vi "command_file__duration.vi"() -> ()   [LabVIEW 2019]
uses:
  Global Variables/global.vi
  Global Variables/Data_Display_global.vi
  Instrument_Setup.vi
panel:
  out "Remaining measurement time of row":string
  out "Measurement ends:":string
  out "Remaining measurement time":string
  out "Measurement Time":string
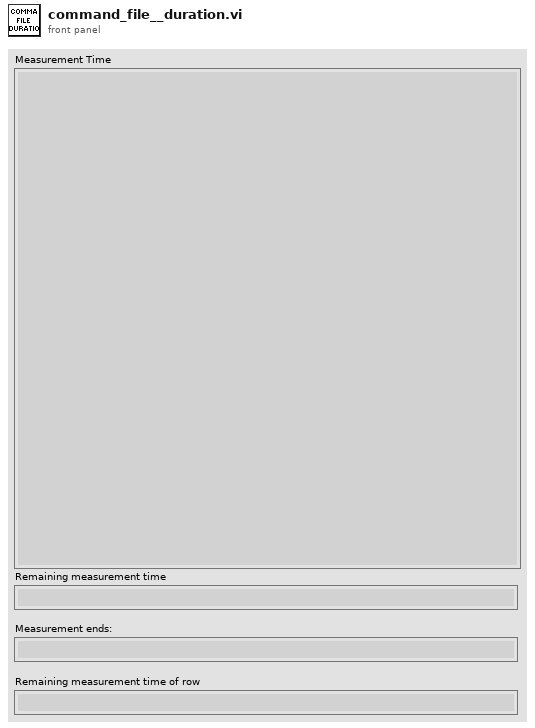
[diagram p1: front panel]
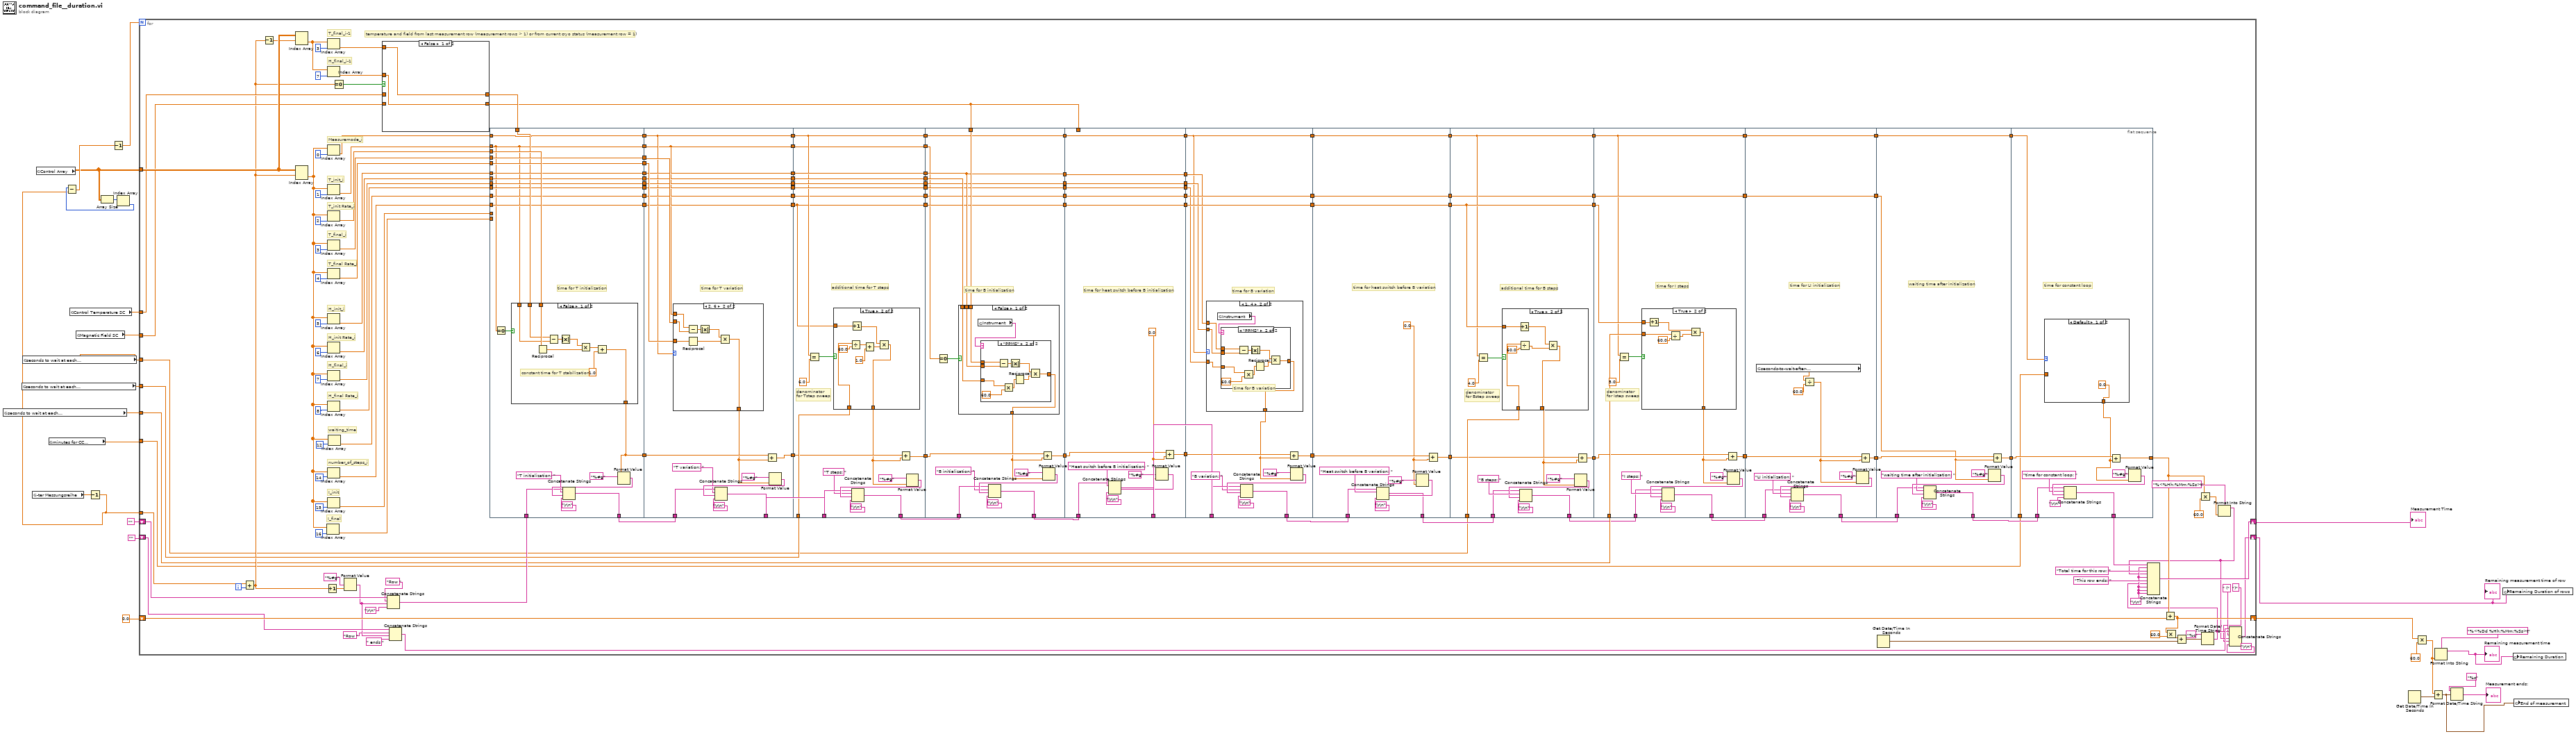
[diagram p0: block diagram]
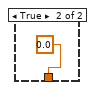
[diagram p3: hidden frame]
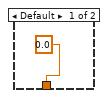
[diagram p4: hidden frame]
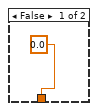
[diagram p5: hidden frame]
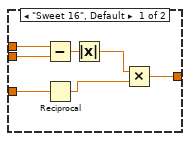
[diagram p6: hidden frame]
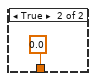
[diagram p7: hidden frame]
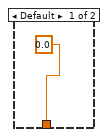
[diagram p8: hidden frame]
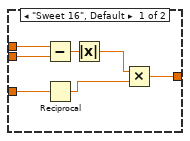
[diagram p9: hidden frame]
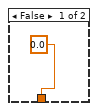
[diagram p10: hidden frame]
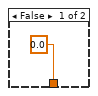
[diagram p11: hidden frame]
diagram:
  n1 = global read "Instrument_Setup.vi" "seconds to wait at each\ncurrent step in a I-step sweep"() -> (w7:dbl)
  n2 = global read "Instrument_Setup.vi" "seconds to wait at each\nfield step in a step sweep"() -> (w8:dbl)
  n3 = global read "Instrument_Setup.vi" "seconds to wait at each\nfield step in a step sweep"() -> (w9:dbl)
  n4 = global read "global.vi" "-ter Messungsreihe"() -> (w4:dbl)
  n5 = global read "global.vi" "Control Array"() -> (w14:dbl[][])
  n6 = global read "Instrument_Setup.vi" "minutes for CC\nto run"() -> (w6:dbl)
  n7 = global read "Data_Display_global.vi" "Control Temperature SC"() -> (w11:dbl)
  n8 = global read "Data_Display_global.vi" "Magnetic Field SC"() -> (w10:dbl)
  n9 = Decrement(x=w4) -> (x-1=w5:dbl)
  n10 = Array Size(array=w14) -> (size(s)=w27:i32[])
  n11 = Index Array(array=w27) -> (element=w22:i32)  [unwired: 1 in]
  n12 = Subtract(x=w22, y=w5) -> (x-y=w23:dbl)
  n13 = Decrement(x=w23) -> (x-1=w26:dbl)
  n14 = for {
    N: w26 -> [_]
    tunnel: w14 -> [w154]
    shift-right: [w130] -> w24
    shift-left: "" -> [w123]
    tunnel: w11 -> [w147]
    tunnel: w10 -> [w146]
    tunnel: w9 -> [w96]
    tunnel: w5 -> [w156]
    tunnel: w8 -> [w135]
    tunnel: w7 -> [w91]
    shift-right: [w71] -> w19
    shift-left: 0.0 -> [w76]
    tunnel: w6 -> [w42]
    shift-right: [w35] -> w2
    shift-left: "" -> [w39]
    i -> [w155]
    w68 = "\r\n"
    # "waiting_time"
    # "I_final"
    # "I_init"
    # "temperature and field from last measurement row (measurement rows > 1) or from current cryo status (measurement row = 1)"
    # "H_final_i-1"
    # "T_final_i-1"
    # "Measuremode_i"
    # "number_of_steps_i"
    # "H_final Rate_i"
    # "H_final_i"
    # "H_init Rate_i"
    # "H_init_i"
    # "T_final Rate_i"
    # "T_final_i"
    # "T_init Rate_i"
    # "T_init_i"
    n15 = Add(x=w156, y=w155) -> (x+y=w121:dbl)
    n16 = Decrement(x=w121) -> (x-1=w153:dbl)
    n17 = Index Array(array=w154, index (row)=w153) -> (element=w150:dbl[])  [unwired: 1 in]
    n18 = Index Array(array=w154, index (row)=w121) -> (element=w60:dbl[])  [unwired: 1 in]
    n19 = Increment(x=w121) -> (x+1=w120:dbl)
    n20 = Index Array(array=w60, index=16) -> (element=w92:dbl)
    n21 = Index Array(array=w150, index=3) -> (element=w149:dbl)
    n22 = Index Array(array=w150, index=7) -> (element=w148:dbl)
    n23 = Index Array(array=w60, index=0) -> (element=w157:dbl)
    n24 = Index Array(array=w60, index=1) -> (element=w172:dbl)
    n25 = Index Array(array=w60, index=2) -> (element=w171:dbl)
    n26 = Index Array(array=w60, index=3) -> (element=w170:dbl)
    n27 = Index Array(array=w60, index=4) -> (element=w169:dbl)
    n28 = Index Array(array=w60, index=5) -> (element=w168:dbl)
    n29 = Index Array(array=w60, index=6) -> (element=w167:dbl)
    n30 = Index Array(array=w60, index=7) -> (element=w166:dbl)
    n31 = Index Array(array=w60, index=8) -> (element=w165:dbl)
    n32 = Index Array(array=w60, index=14) -> (element=w160:dbl)
    n33 = Index Array(array=w60, index=15) -> (element=w93:dbl)
    n34 = Index Array(array=w60, index=12) -> (element=w59:dbl)
    n35 = Equal To 0?(x=w121) -> (x = 0?=w145:bool)
    n36 = Format Value(format string="%#g", value (0)=w120) -> (output string=w37:string)  [unwired: 1 in]
    n37 = case shown="False" w145 {
      tunnel: w149 -> [w181 _]
      tunnel: w148 -> [w182 _]
      tunnel: w147 -> [_ w184]
      tunnel: w146 -> [_ w183]
      tunnel: [w181 w184] -> w144
      tunnel: [w182 w183] -> w109
      frame False {
      }
      frame True {
      }
    }
    n38 = Concatenate Strings(w123, "Row ", w37, "\r\n") -> (w122:string)
    n39 = Concatenate Strings(w39, "Row ", w37, " ends ") -> (w32:string)
    n40 = flat-sequence {
      tunnel: w172 -> [w185]
      tunnel: w171 -> [w204]
      tunnel: w122 -> [w191]
      tunnel: [w202] -> w161
      tunnel: w170 -> [w199]
      tunnel: w169 -> [w198]
      tunnel: w168 -> [w197]
      tunnel: w167 -> [w196]
      tunnel: w166 -> [w193]
      tunnel: w165 -> [w192]
      tunnel: [w185] -> w164
      tunnel: [w199] -> w163
      tunnel: [w198] -> w162
      tunnel: w160 -> [w194]
      tunnel: [w197] -> w159
      tunnel: [w196] -> w158
      tunnel: w157 -> [w186]
      tunnel: w144 -> [w195]
      tunnel: [w186] -> w136
      tunnel: [w194] -> w133
      tunnel: [w193] -> w129
      tunnel: [w192] -> w124
      tunnel: w93 -> [_]
      tunnel: w92 -> [_]
      tunnel: [w189] -> w86
      tunnel: w59 -> [w188]
      tunnel: [w188] -> w49
      tunnel: w164 -> [w215]
      tunnel: w163 -> [w230]
      tunnel: w162 -> [w229]
      tunnel: [w228] -> w132
      tunnel: w161 -> [w222]
      tunnel: w159 -> [w227]
      tunnel: [w227] -> w141
      tunnel: [w226] -> w139
      tunnel: w158 -> [w226]
      tunnel: [w216] -> w137
      tunnel: w136 -> [w216]
      tunnel: [w225] -> w134
      tunnel: w133 -> [w225]
      tunnel: w129 -> [w224]
      tunnel: [w224] -> w127
      tunnel: [w223] -> w125
      tunnel: w124 -> [w223]
      tunnel: w86 -> [w220]
      tunnel: [w218] -> w85
      tunnel: [w217] -> w50
      tunnel: w49 -> [w217]
      tunnel: [w215] -> w40
      tunnel: w141 -> [w261]
      tunnel: [w261] -> w140
      tunnel: w139 -> [w260]
      tunnel: [w260] -> w138
      tunnel: w137 -> [w248]
      tunnel: w135 -> [w257]
      tunnel: w134 -> [w247]
      tunnel: w132 -> [w250]
      tunnel: [w253] -> w131
      tunnel: [w252] -> w128
      tunnel: w127 -> [w252]
      tunnel: [w251] -> w126
      tunnel: w125 -> [w251]
      tunnel: [w248] -> w102
      tunnel: [w247] -> w97
      tunnel: w85 -> [w246]
      tunnel: [w244] -> w84
      tunnel: [w243] -> w51
      tunnel: w50 -> [w243]
      tunnel: [w242] -> w41
      tunnel: w40 -> [w242]
      tunnel: w131 -> [w280]
      tunnel: [w286] -> w111
      tunnel: w140 -> [w283]
      tunnel: w138 -> [w285]
      tunnel: w109 -> [w284]
      tunnel: [w283] -> w117
      tunnel: [w282] -> w115
      tunnel: w128 -> [w282]
      tunnel: [w281] -> w113
      tunnel: w126 -> [w281]
      tunnel: [w278] -> w103
      tunnel: w102 -> [w278]
      tunnel: [w277] -> w98
      tunnel: w97 -> [w277]
      tunnel: w84 -> [w276]
      tunnel: [w274] -> w83
      tunnel: [w273] -> w52
      tunnel: w51 -> [w273]
      tunnel: w41 -> [w271]
      tunnel: w117 -> [w320]
      tunnel: [w320] -> w116
      tunnel: w115 -> [w326]
      tunnel: [w326] -> w114
      tunnel: w113 -> [w325]
      tunnel: [w325] -> w112
      tunnel: w111 -> [w322]
      tunnel: [w321] -> w110
      tunnel: w109 -> [_]
      tunnel: [w317] -> w104
      tunnel: w103 -> [w317]
      tunnel: [w316] -> w99
      tunnel: w98 -> [w316]
      tunnel: w83 -> [w315]
      tunnel: [w313] -> w82
      tunnel: [w312] -> w53
      tunnel: w52 -> [w312]
      tunnel: w116 -> [w331]
      tunnel: w114 -> [w330]
      tunnel: w112 -> [w329]
      tunnel: w110 -> [w337]
      tunnel: [w339] -> w108
      tunnel: [w327] -> w105
      tunnel: w104 -> [w327]
      tunnel: [w335] -> w100
      tunnel: w99 -> [w335]
      tunnel: w82 -> [w334]
      tunnel: [w333] -> w81
      tunnel: [w332] -> w54
      tunnel: w53 -> [w332]
      tunnel: w108 -> [w371]
      tunnel: [w370] -> w107
      tunnel: [w369] -> w106
      tunnel: w105 -> [w369]
      tunnel: [w368] -> w101
      tunnel: w100 -> [w368]
      tunnel: w81 -> [w367]
      tunnel: [w365] -> w80
      tunnel: [w364] -> w55
      tunnel: w54 -> [w364]
      tunnel: w107 -> [w384]
      tunnel: [w383] -> w90
      tunnel: w106 -> [w380]
      tunnel: w101 -> [w381]
      tunnel: w96 -> [w382]
      tunnel: [w381] -> w89
      tunnel: [w380] -> w88
      tunnel: w80 -> [w379]
      tunnel: [w377] -> w79
      tunnel: [w376] -> w56
      tunnel: w55 -> [w376]
      tunnel: w91 -> [w405]
      tunnel: w90 -> [w408]
      tunnel: [w407] -> w87
      tunnel: w89 -> [w406]
      tunnel: w88 -> [w398]
      tunnel: w79 -> [w402]
      tunnel: [w400] -> w78
      tunnel: [w399] -> w57
      tunnel: w56 -> [w399]
      tunnel: [w398] -> w43
      tunnel: w87 -> [w428]
      tunnel: [w427] -> w62
      tunnel: w78 -> [w426]
      tunnel: [w425] -> w63
      tunnel: [w424] -> w58
      tunnel: w57 -> [w424]
      tunnel: [w423] -> w44
      tunnel: w43 -> [w423]
      tunnel: w63 -> [w437]
      tunnel: w62 -> [w436]
      tunnel: [w435] -> w46
      tunnel: w58 -> [w434]
      tunnel: [w438] -> w48
      tunnel: [w433] -> w45
      tunnel: w44 -> [w433]
      tunnel: [w453] -> w64
      tunnel: w48 -> [w452]
      tunnel: [w448] -> w47
      tunnel: w46 -> [w447]
      tunnel: w45 -> [w445]
      tunnel: w42 -> [w444]
      frame #0 {
        # "time for T initialization"
        n41 = Equal To 0?(x=w185) -> (x = 0?=w187:bool)
        n42 = case shown="False" w187 {
          tunnel: w204 -> [w212 _]
          tunnel: w185 -> [w209 _]
          tunnel: w195 -> [w206 _]
          tunnel: [w205 0.0] -> w189
          frame False {
            # "constant time for T stabilization"
            n43 = Reciprocal(x=w212) -> (1/x=w211:dbl)
            n44 = Subtract(x=w206, y=w209) -> (x-y=w213:dbl)
            n45 = Absolute Value(x=w213) -> (abs(x)=w210:dbl)
            n46 = Multiply(x=w210, y=w211) -> (x*y=w208:dbl)
            n47 = Add(x=w208, y=1.0) -> (x+y=w205:dbl)
          }
          frame True {
          }
        }
        n48 = Format Value(format string="%#g", value (0)=w189) -> (output string=w200:string)  [unwired: 1 in]
        n49 = Concatenate Strings(w191, "T initialization: ", w200, "\r\n") -> (w202:string)
      }
      frame #1 {
        # "time for T variation"
        n50 = case shown="2, 6" w216 {
          tunnel: w215 -> [_ w238]
          tunnel: w230 -> [_ w237]
          tunnel: w229 -> [_ w236]
          tunnel: [0.0 w235] -> w219
          frame Default {
          }
          frame 2, 6 {
            n51 = Subtract(x=w238, y=w237) -> (x-y=w241:dbl)
            n52 = Reciprocal(x=w236) -> (1/x=w240:dbl)
            n53 = Absolute Value(x=w241) -> (abs(x)=w239:dbl)
            n54 = Multiply(x=w239, y=w240) -> (x*y=w235:dbl)
          }
        }
        n55 = Add(x=w220, y=w219) -> (x+y=w218:dbl)
        n56 = Format Value(format string="%#g", value (0)=w219) -> (output string=w231:string)  [unwired: 1 in]
        n57 = Concatenate Strings(w222, "T variation: ", w231, "\r\n") -> (w228:string)
      }
      frame #2 {
        # "denominator\nfor Tstep sweep"
        # "additional time for T steps"
        n58 = Equal?(x=w248, y=6.0) -> (x = y?=w258:bool)
        n59 = case shown="True" w258 {
          tunnel: w247 -> [_ w264]
          tunnel: w257 -> [_ w270]
          tunnel: [0.0 w265] -> w245
          frame False {
          }
          frame True {
            n60 = Divide(x=w270, y=60.0) -> (x/y=w268:dbl)
            n61 = Increment(x=w264) -> (x+1=w263:dbl)
            n62 = Add(x=w268, y=1.0) -> (x+y=w266:dbl)
            n63 = Multiply(x=w263, y=w266) -> (x*y=w265:dbl)
          }
        }
        n64 = Add(x=w246, y=w245) -> (x+y=w244:dbl)
        n65 = Format Value(format string="%#g", value (0)=w245) -> (output string=w254:string)  [unwired: 1 in]
        n66 = Concatenate Strings(w250, "T steps: ", w254, "\r\n") -> (w253:string)
      }
      frame #3 {
        # "time for B initialization"
        n67 = Equal To 0?(x=w271) -> (x = 0?=w272:bool)
        n68 = case shown="False" w272 {
          tunnel: w285 -> [w294 _]
          tunnel: w284 -> [w293 _]
          tunnel: w283 -> [w292 _]
          tunnel: [w291 0.0] -> w275
          frame False {
            n69 = global read "Instrument_Setup.vi" "Instrument"() -> (w290:string)
            n70 = case shown="\"PPMS\"" w290 {
              tunnel: w294 -> [w298 w303]
              tunnel: w293 -> [w297 w306]
              tunnel: w292 -> [w296 w305]
              tunnel: [w295 w307] -> w291
              frame "Sweet 16", Default {
                n71 = Subtract(x=w297, y=w296) -> (x-y=w301:dbl)
                n72 = Reciprocal(x=w298) -> (1/x=w300:dbl)
                n73 = Absolute Value(x=w301) -> (abs(x)=w299:dbl)
                n74 = Multiply(x=w299, y=w300) -> (x*y=w295:dbl)
              }
              frame "PPMS" {
                n75 = Subtract(x=w306, y=w305) -> (x-y=w310:dbl)
                n76 = Multiply(x=w303, y=60.0) -> (x*y=w302:dbl)
                n77 = Absolute Value(x=w310) -> (abs(x)=w308:dbl)
                n78 = Reciprocal(x=w302) -> (1/x=w309:dbl)
                n79 = Multiply(x=w308, y=w309) -> (x*y=w307:dbl)
              }
            }
          }
          frame True {
          }
        }
        n80 = Add(x=w276, y=w275) -> (x+y=w274:dbl)
        n81 = Format Value(format string="%#g", value (0)=w275) -> (output string=w287:string)  [unwired: 1 in]
        n82 = Concatenate Strings(w280, "B initialization: ", w287, "\r\n") -> (w286:string)
      }
      frame #4 {
        w314 = 0.0
        # "time for heat switch before B initialization"
        n83 = Format Value(format string="%#g", value (0)=w314) -> (output string=w318:string)  [unwired: 1 in]
        n84 = Concatenate Strings(w322, "Heat switch before B initialization: ", w318, "\r\n") -> (w321:string)
        n85 = Add(x=w315, y=w314) -> (x+y=w313:dbl)
      }
      frame #5 {
        # "time for B variation"
        # "time for B variation"
        n86 = case shown="1, 4" w327 {
          tunnel: w331 -> [_ w347]
          tunnel: w330 -> [_ w345]
          tunnel: w329 -> [_ w344]
          tunnel: [0.0 w343] -> w328
          frame Default {
          }
          frame 1, 4 {
            n87 = global read "Instrument_Setup.vi" "Instrument"() -> (w346:string)
            n88 = case shown="\"PPMS\"" w346 {
              tunnel: w344 -> [w351 w356]
              tunnel: w347 -> [w350 w359]
              tunnel: w345 -> [w349 w358]
              tunnel: [w348 w360] -> w343
              frame "Sweet 16", Default {
                n89 = Subtract(x=w350, y=w349) -> (x-y=w354:dbl)
                n90 = Reciprocal(x=w351) -> (1/x=w353:dbl)
                n91 = Absolute Value(x=w354) -> (abs(x)=w352:dbl)
                n92 = Multiply(x=w352, y=w353) -> (x*y=w348:dbl)
              }
              frame "PPMS" {
                n93 = Subtract(x=w359, y=w358) -> (x-y=w363:dbl)
                n94 = Multiply(x=w356, y=60.0) -> (x*y=w355:dbl)
                n95 = Absolute Value(x=w363) -> (abs(x)=w361:dbl)
                n96 = Reciprocal(x=w355) -> (1/x=w362:dbl)
                n97 = Multiply(x=w361, y=w362) -> (x*y=w360:dbl)
              }
            }
          }
        }
        n98 = Add(x=w334, y=w328) -> (x+y=w333:dbl)
        n99 = Format Value(format string="%#g", value (0)=w328) -> (output string=w340:string)  [unwired: 1 in]
        n100 = Concatenate Strings(w337, "B variation: ", w340, "\r\n") -> (w339:string)
      }
      frame #6 {
        w366 = 0.0
        # "time for heat switch before B variation"
        n101 = Format Value(format string="%#g", value (0)=w366) -> (output string=w372:string)  [unwired: 1 in]
        n102 = Concatenate Strings(w371, "Heat switch before B variation: ", w372, "\r\n") -> (w370:string)
        n103 = Add(x=w367, y=w366) -> (x+y=w365:dbl)
      }
      frame #7 {
        # "denominator\nfor Bstep sweep"
        # "additional time for B steps"
        n104 = Equal?(x=w380, y=4.0) -> (x = y?=w386:bool)
        n105 = case shown="True" w386 {
          tunnel: w381 -> [_ w393]
          tunnel: w382 -> [_ w397]
          tunnel: [0.0 w395] -> w378
          frame False {
          }
          frame True {
            n106 = Increment(x=w393) -> (x+1=w392:dbl)
            n107 = Divide(x=w397, y=60.0) -> (x/y=w394:dbl)
            n108 = Multiply(x=w392, y=w394) -> (x*y=w395:dbl)
          }
        }
        n109 = Format Value(format string="%#g", value (0)=w378) -> (output string=w389:string)  [unwired: 1 in]
        n110 = Concatenate Strings(w384, "B steps: ", w389, "\r\n") -> (w383:string)
        n111 = Add(x=w379, y=w378) -> (x+y=w377:dbl)
      }
      frame #8 {
        # "denominator\nfor Istep sweep"
        # "time for I steps"
        n112 = Equal?(x=w398, y=5.0) -> (x = y?=w403:bool)
        n113 = case shown="True" w403 {
          tunnel: w406 -> [_ w415]
          tunnel: w405 -> [_ w417]
          tunnel: [0.0 w416] -> w401
          frame False {
          }
          frame True {
            n114 = Increment(x=w415) -> (x+1=w414:dbl)
            n115 = Divide(x=w417, y=60.0) -> (x/y=w419:dbl)
            n116 = Multiply(x=w414, y=w419) -> (x*y=w416:dbl)
          }
        }
        n117 = Add(x=w402, y=w401) -> (x+y=w400:dbl)
        n118 = Format Value(format string="%#g", value (0)=w401) -> (output string=w411:string)  [unwired: 1 in]
        n119 = Concatenate Strings(w408, "I steps: ", w411, "\r\n") -> (w407:string)
      }
      frame #9 {
        # "time for LI initialization"
        n120 = global read "Instrument_Setup.vi" "seconds-to-wait-after-\nLock-In-initialization"() -> (w421:dbl)
        n121 = Divide(x=w421, y=60.0) -> (x/y=w422:dbl)
        n122 = Format Value(format string="%#g", value (0)=w422) -> (output string=w431:string)  [unwired: 1 in]
        n123 = Concatenate Strings(w428, "LI initialization: ", w431, "\r\n") -> (w427:string)
        n124 = Add(x=w426, y=w422) -> (x+y=w425:dbl)
      }
      frame #10 {
        # "waiting time after initialization"
        n125 = Format Value(format string="%#g", value (0)=w434) -> (output string=w440:string)  [unwired: 1 in]
        n126 = Concatenate Strings(w436, "waiting time after initialization: ", w440, "\r\n") -> (w435:string)
        n127 = Add(x=w437, y=w434) -> (x+y=w438:dbl)
      }
      frame #11 {
        # "time for constant loop"
        n128 = case shown="Default" w445 {
          tunnel: [0.0 w455] -> w446
          tunnel: w444 -> [_ w455]
          frame Default {
          }
          frame 3 {
          }
        }
        n129 = Add(x=w452, y=w446) -> (x+y=w453:dbl)
        n130 = Format Value(format string="%#g", value (0)=w446) -> (output string=w450:string)  [unwired: 1 in]
        n131 = Concatenate Strings(w447, "time for constant loop: ", w450, "\r\n") -> (w448:string)
      }
    }
    n132 = Get Date/Time In Seconds() -> (seconds since 1Jan1904=w73:timestamp)
    n133 = Add(x=w64, y=w76) -> (x+y=w71:dbl)
    n134 = Multiply(x=w71, y=60.0) -> (x*y=w70:dbl)
    n135 = Add(x=w70, y=w73) -> (x+y=w74:timestamp)
    n136 = Multiply(x=w64, y=60.0) -> (x*y=w65:dbl)
    n137 = Format Date/Time String(time format string (%c)="%c", seconds (now)=w74) -> (date/time string=w31:string)  [unwired: 1 in]
    n138 = Format Into String(format string="%<%Hh:%Mm:%Ss>t", w65) -> (resulting string=w29:string)  [unwired: 2 in, 1 out]
    n139 = Concatenate Strings(w47, w68, "Total time for this row: ", w29, w68, "This row ends: ", w31, w68, w68, w68) -> (w130:string)
    n140 = Concatenate Strings(w32, w31, " (", w29, ")", "\r\n") -> (w35:string)
  }
  "Measurement Time" <- w24
  "Remaining measurement time of row" <- w2
  n141 = Get Date/Time In Seconds() -> (seconds since 1Jan1904=w16:timestamp)
  n142 = Multiply(x=w19, y=60.0) -> (x*y=w17:dbl)
  n143 = Add(x=w17, y=w16) -> (x+y=w1:timestamp)
  n144 = Format Into String(format string="%<%Dd %Hh:%Mm:%Ss>t", w17) -> (resulting string=w13:string)  [unwired: 2 in, 1 out]
  "Remaining measurement time" <- w13
  n145 = Format Date/Time String(time format string (%c)="%c", seconds (now)=w1) -> (date/time string=→"Measurement ends:":string)  [unwired: 1 in]
  n146 = global write "Data_Display_global.vi" "Remaining Duration of rows"(w2) -> ()
  n147 = global write "Data_Display_global.vi" "Remaining Duration"(w13) -> ()
  n148 = global write "Data_Display_global.vi" "End of measurement"(w1) -> ()
